vi "labourShippingDiscount.vi"(0 "reference in":refnum<class "excelFile.lvclass">, 2 "TSR_details":T1={"Company/Institution:"="", "Address:"="", "Department:"="", "City:"="", "Post Code:"="", "Country:"="", "Contact:"="", "Ref:"="", "Issue description:"="", "Actions:"="", "TYPE:"="Repair", "Shipping:"=0, "Discount:"=0, "dataIN"=[], "Device type:"="microQuark", "Serial Number:"="", "PMC number:"="", "Labour Hours:"=0.0, "Service Location:"=FALSE, "start_hour"="", "end_hour"="", "o2_exp_date"="", "GST"=TRUE}, 5 "error in (no error)":errorcluster) -> (14 "reference out":refnum<class "excelFile.lvclass">, 19 "error out":errorcluster)   [LabVIEW 2016, in "excelFile.lvclass"]
uses:
  excelFile.lvclass
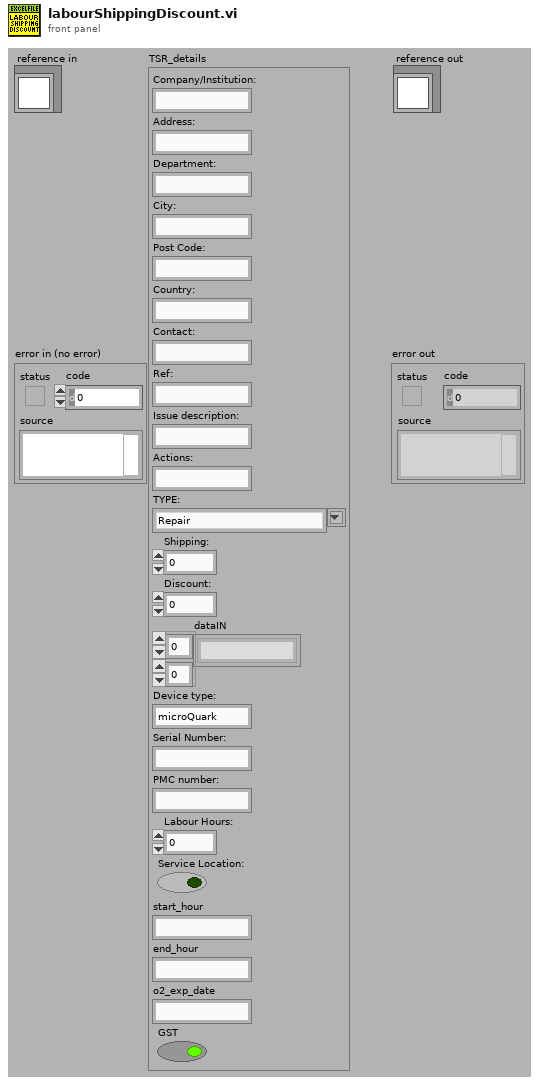
[diagram p1: front panel]
types:
  T1 = cluster{"Company/Institution:":string, "Address:":string, "Department:":string, "City:":string, "Post Code:":string, "Country:":string, "Contact:":string, "Ref:":string, "Issue description:":string, "Actions:":string, "TYPE:":string, "Shipping:":i32, "Discount:":i32, "dataIN":string[][], "Device type:":string, "Serial Number:":string, "PMC number:":string, "Labour Hours:":dbl, "Service Location:":bool, "start_hour":string, "end_hour":string, "o2_exp_date":string, "GST":bool}
  T2 = typedef "excelFile.lvclass/ObjectAttributesRef.ctl" = refnum<data-value>
  T3 = typedef "excelFile.lvclass/ObjectAttributes.ctl" = cluster{"MyAttribute":dbl, "path":string, "Refnum Excel":cluster{"Excel._Application":refnum<k7>, "Workbooks":refnum<k7>, "Open":refnum<k7>}, "data":string[][][], "save":bool, "fileType":T4, "rowsColor":u32[], "python_ref":refnum<class "python.lvclass">, "items_rows":i32[], "excel_range":i32[][], "TSR":cluster{"number":string, "TSR_path":path, "service_path":path, "email_to":string}, "excel_already_opened?":bool, "file_already_opened?":bool, "excel_protected_opened?":bool, "Refnum Cluster Worksheets":cluster{"Excel._Application":refnum<k7>, "Workbooks":refnum<k7>, "Open":refnum<k7>, "Worksheets":refnum<k7>, "Excel._Worksheet":refnum<k7>}, "#_rows_defective":i32, "#_rows_spare":i32}
  T4 = typedef "excelFile.lvclass/fileType.ctl" = enum16{"devices", "items", "partsTracking", "TSR"}
  T5 = cluster{"Excel._Application":refnum<k7>, "Workbooks":refnum<k7>, "Open":refnum<k7>, "Worksheets":refnum<k7>, "Excel._Worksheet":refnum<k7>}
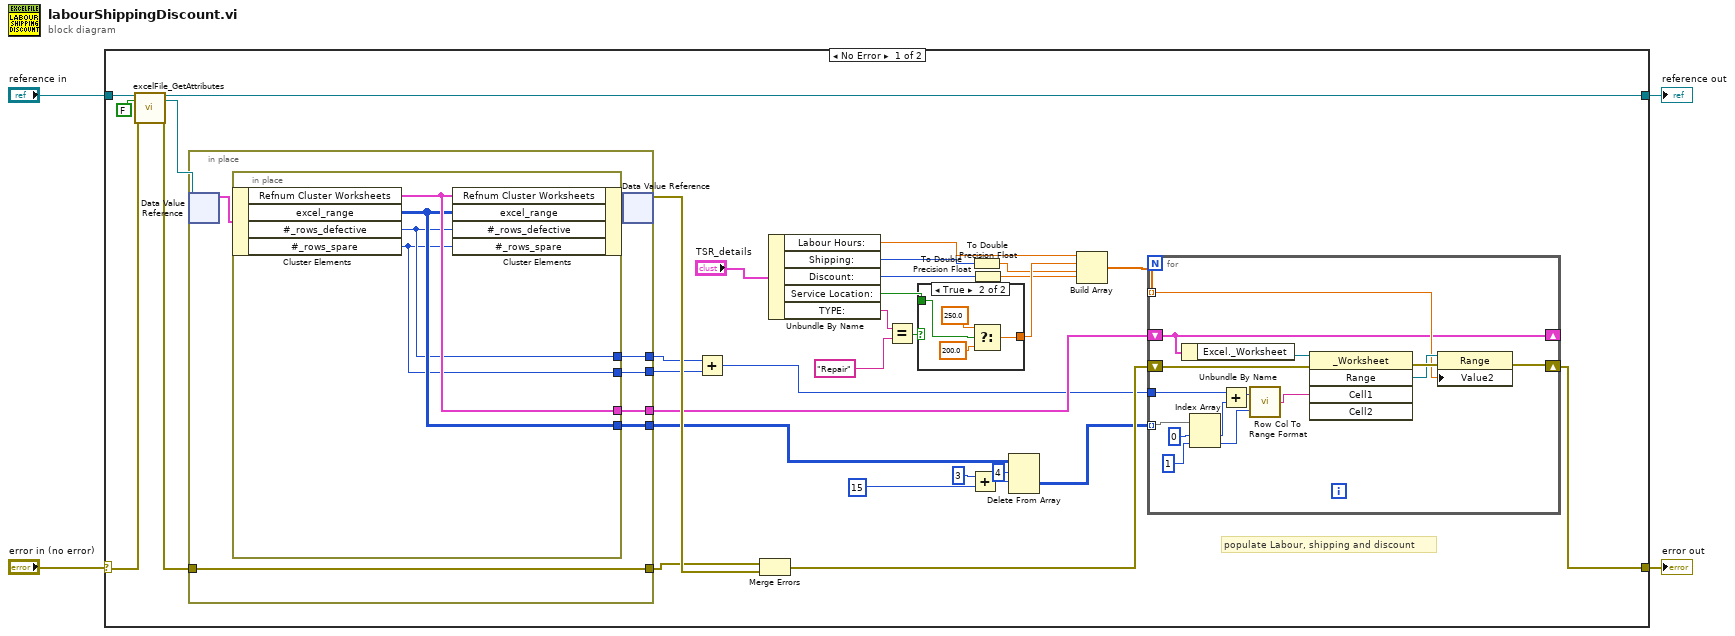
[diagram p0: block diagram]
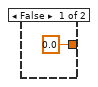
[diagram p2: hidden frame]
diagram:
  n1 = case shown="No Error" "error in (no error)" {
    selector: "error in (no error)" -> [w33 w69]
    tunnel: [w18 w69] -> w3
    tunnel: [w31 w68] -> w1
    tunnel: "reference in" -> [w35 w68]
    frame No Error {
      # "populate Labour, shipping and discount"
      n2 = call "excelFile_GetAttributes.vi"("reference in"=w35, "return data? (T)"=FALSE, "error in (no error)"=w33) -> ("reference out"=w31:refnum<class "excelFile.lvclass">, "attributes ref"=w30:T2, "error out"=w32:errorcluster)  [unwired: 13 in, 1 out]
      n3 = in-place {
        in-place-border: w32 -> [w61]
        in-place-border: [w61] -> w20
        in-place-border: [w60] -> w19
        in-place-border: [w59] -> w13
        in-place-border: [w58] -> w11
        in-place-border: [w57] -> w10
        n4 = in-place-dvr #1(w30) -> (w62:T3)  [unwired: 1 out]
        n5 = in-place {
          in-place-border: [w67] -> w60
          in-place-border: [w66] -> w59
          in-place-border: [w65] -> w58
          in-place-border: [w64] -> w57
          n6 = in-place-cluster #2(w62) -> ("Refnum Cluster Worksheets"=w67:T5, "excel_range"=w66:i32[][], "#_rows_defective"=w65:i32, "#_rows_spare"=w64:i32)
          n7 = in-place-cluster #2("Refnum Cluster Worksheets"=w67, "excel_range"=w66, "#_rows_defective"=w65, "#_rows_spare"=w64) -> (w63:T3)
        }
        n8 = in-place-dvr #1(w63) -> (w36:errorcluster)  [unwired: 1 out]
      }
      n9 = Add(x=w11, y=w10) -> (x+y=w9:i32)
      n10 = Merge Errors(w20, w36) -> (w21:errorcluster)
      n11 = Unbundle By Name("TSR_details") -> ("Labour Hours:"=w29:dbl, "Shipping:"=w24:i32, "Discount:"=w26:i32, "Service Location:"=w28:bool, "TYPE:"=w7:string)
      n12 = Equal?(x=w7, y="Repair") -> (x = y?=w5:bool)
      n13 = case shown="True" w5 {
        tunnel: w28 -> [_ w41]
        tunnel: [0.0 w38] -> w25
        frame False {
        }
        frame True {
          n14 = Select(t=250.0, s=w41, f=200.0) -> (s? t:f=w38:dbl)
        }
      }
      n15 = Add(x=3, y=15) -> (x+y=w17:i32)
      n16 = To Double Precision Float(number=w24) -> (double precision float=w23:dbl)
      n17 = To Double Precision Float(number=w26) -> (double precision float=w22:dbl)
      n18 = Delete From Array(array=w13, length=4 ("index"), index (row)=w17) -> (deleted portion=w12:i32[][])  [unwired: 1 in, 1 out]
      n19 = Build Array(w29, w25, w23, w22) -> (w27:dbl[])
      n20 = for {
        shift-right: [w45] -> w18
        shift-left: w21 -> [w47]
        shift-right: [w44] -> _
        shift-left: w19 -> [w44]
        tunnel: w12 -> [w52] mode=indexing
        tunnel: w27 -> [w46] mode=indexing
        tunnel: w9 -> [w42]
        n21 = Unbundle By Name(w44) -> ("Excel._Worksheet"=w53:refnum<k7>)
        n22 = Index Array(array=w52, index #1=0 ("index"), index #2=1 ("index")) -> (element #1=w49:i32, element #2=w48:i32)
        n23 = Add(x=w42, y=w49) -> (x+y=w43:i32)
        n24 = call <userlib>:"Row Col To Range Format.vi"("Column"=w48, "Row"=w43) -> ("Output String"=w56:string)
        n25 = invoke class="_Worksheet" method="Range"(reference=w53, error in=w47, "Cell1"=w56) -> (error out=w55:errorcluster, "Range"=w54:refnum<k7>)  [unwired: 2 in, 3 out]
        n26 = property class="Range"(reference=w54, error in=w55, "Value2"=w46) -> (error out=w45:errorcluster)  [unwired: 1 out]
      }
    }
    frame Error {
    }
  }
  "error out" <- w3
  "reference out" <- w1
